vi "Status Setpoint.vi"(0 "VISA resource name":refnum<visa-resource-name>, 7 "Loop (0: 1)":u16(ring) items=["1", "2"], 11 "error in (no error)":errorcluster) -> (4 "VISA resource name out":refnum<visa-resource-name>, 8 "Setpoint":dbl min=-273.0 max=300000.0 step=1e-05 format="%.5f", 15 "error out":errorcluster)   [LabVIEW 2019, in "Lake Shore Cryotronics 340.lvlib"]
doc: "This VI indicates a control loop's setpoint."
uses:
  Lake Shore Cryotronics 340.lvlib
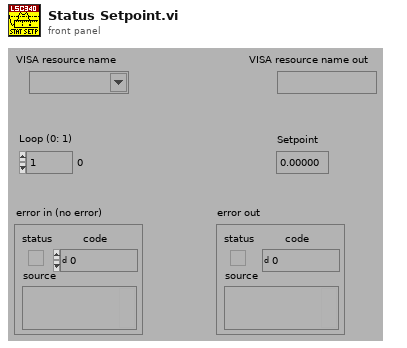
[diagram p1: front panel]
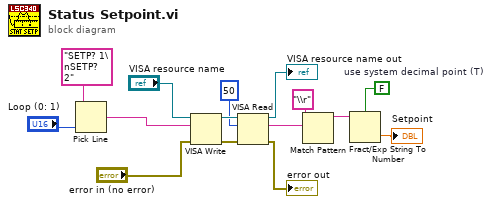
[diagram p0: block diagram]
diagram:
  w1 = FALSE  # use system decimal point (T)
  n1 = Pick Line(multi-line string="SETP? 1\nSETP? 2", line index="Loop (0: 1)") -> (output string=w6:string)  [unwired: 1 in]
  n2 = VISA Write(VISA resource name="VISA resource name", write buffer=w6, error in (no error)="error in (no error)") -> (VISA resource name out=w12:refnum<visa-resource-name>, error out=w11:errorcluster)  [unwired: 1 out]
  n3 = VISA Read(VISA resource name=w12, byte count=50, error in (no error)=w11) -> (VISA resource name out=→"VISA resource name out":refnum<visa-resource-name>, read buffer=w9:string, error out=→"error out":errorcluster)  [unwired: 1 out]
  n4 = Match Pattern(string=w9, regular expression="\\r") -> (before substring=w15:string)  [unwired: 1 in, 3 out]
  n5 = Fract/Exp String To Number(use system decimal point (T)=w1, string=w15) -> (number=→"Setpoint":dbl)  [unwired: 2 in, 1 out]
